vi "Add Tree Nodes.vi"(6 "App Ref":refnum<vi>, 7 "Root path":string, 8 "Event Types":T1[](array[typedef]), 9 "map ref in":map{string, refnum<vi>}(c390), 10 "DQMH Lib In":refnum<vi>, 11 "Tree Map in":T2) -> (1 "map ref out":map{string, refnum<vi>}(c390), 3 "Tree Map out":T2)   [LabVIEW 2019, in "Panther Dashboard.lvlib"]
uses:
  Panther Dashboard.lvlib
  <vilib>/National Instruments/Tree Map/Tree Map Data.ctl
  Event types--enum.ctl
  <vilib>/Delacor/Delacor QMH/Libraries/Scripting API/DQMH_Scripting API.lvlib
  <vilib>/National Instruments/Tree Map/Tree Map.lvlib
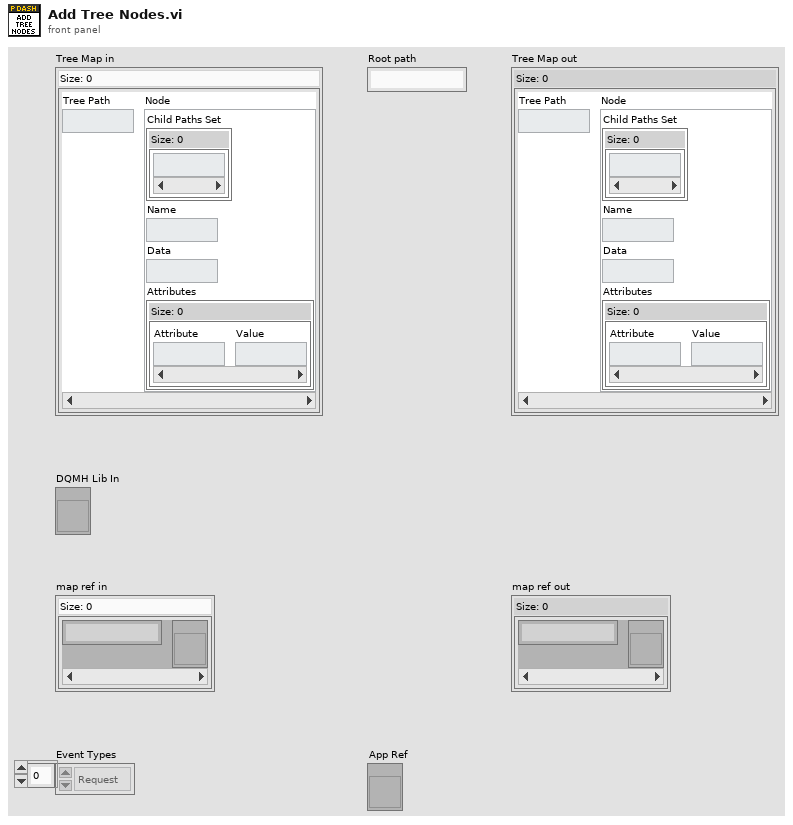
[diagram p1: front panel]
types:
  T1 = typedef "Panther Dashboard.lvlib/Event types--enum.ctl" = enum16{"Request", "Request and Wait for Reply", "Broadcast"}
  T2 = typedef "Tree Map.lvlib/Tree Map Data.ctl" = map{string, cluster{"Child Paths Set":set{string}, "Name":string, "Data":string, "Attributes":map{string, string}}}
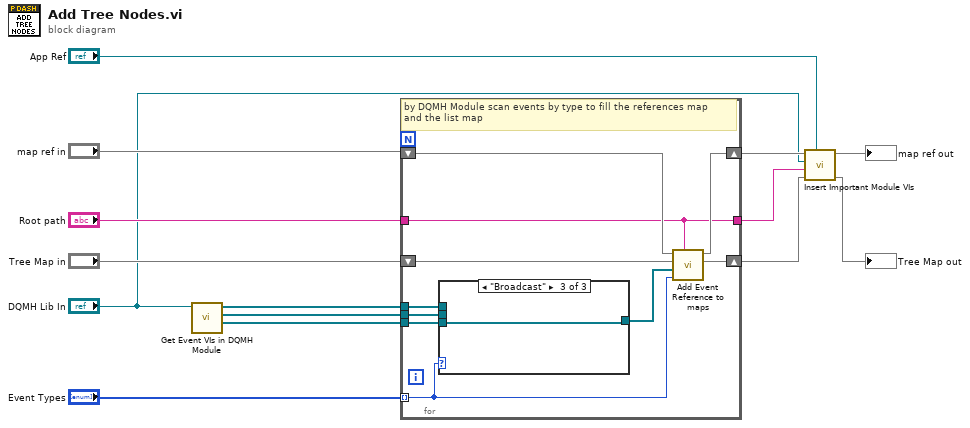
[diagram p0: block diagram]
diagram:
  n1 = call <vilib>:"Get Event VIs in DQMH Module.vi"("DQMH Module"="DQMH Lib In") -> ("Broadcast Event VIs"=w11:refnum<vi>[], "Request and Wait for Reply Event VIs"=w12:refnum<vi>[], "Request Event VIs"=w13:refnum<vi>[])  [unwired: 7 in, 1 out]
  n2 = for {
    tunnel: "Event Types" -> [w16] mode=indexing
    shift-right: [w21] -> w9
    shift-left: "map ref in" -> [w20]
    shift-right: [w22] -> w3
    shift-left: "Tree Map in" -> [w19]
    tunnel: w13 -> [w24]
    tunnel: w12 -> [w18]
    tunnel: w11 -> [w23]
    tunnel: "Root path" -> [w15]
    tunnel: [w15] -> w1
    # "by DQMH Module scan events by type to fill the references map\nand the list map"
    n3 = case shown="\"Broadcast\"" w16 {
      tunnel: w24 -> [w25 _ _]
      tunnel: w23 -> [_ _ w27]
      tunnel: w18 -> [_ w26 _]
      tunnel: [w25 w26 w27] -> w17
      frame "Request" {
      }
      frame "Request and Wait for Reply" {
      }
      frame "Broadcast" {
      }
    }
    n4 = call "Add Event Reference to maps.vi"("New Node Path"=w15, "Event type"=w16, "Event VIs"=w17, "Tree Map in"=w19, "map ref in"=w20) -> ("Tree Map out"=w22:T2, "map ref out"=w21:map{string, refnum<vi>})  [unwired: 5 in]
  }
  n5 = call "Insert Important Module VIs.vi"("Application in"="App Ref", "Tree Map in"=w3, "Root path"=w1, "DQMH Lib In"="DQMH Lib In", "map ref in in"=w9) -> ("Tree Map Out"=→"Tree Map out":T2, "map ref out"=→"map ref out":map{string, refnum<vi>})  [unwired: 5 in]
